vi "Handle Debug Data.vi"(8 "error in (no error)":errorcluster, 10 "Debug Data.lvclass":refnum<class "Debug Data.lvclass">, 11 "Debug Data Event In":refnum<class "Mock Data Listener.lvclass">) -> (0 "error out":errorcluster, 3 "Debug Data Event Out":refnum<class "Mock Data Listener.lvclass">)   [LabVIEW 2020, in "Mock Data Listener.lvclass"]
uses:
  Mock Data Listener.lvclass
  Debug Data/Debug Data.lvclass
  Mock Data Listener.lvclass/Mock Data Listener.ctl
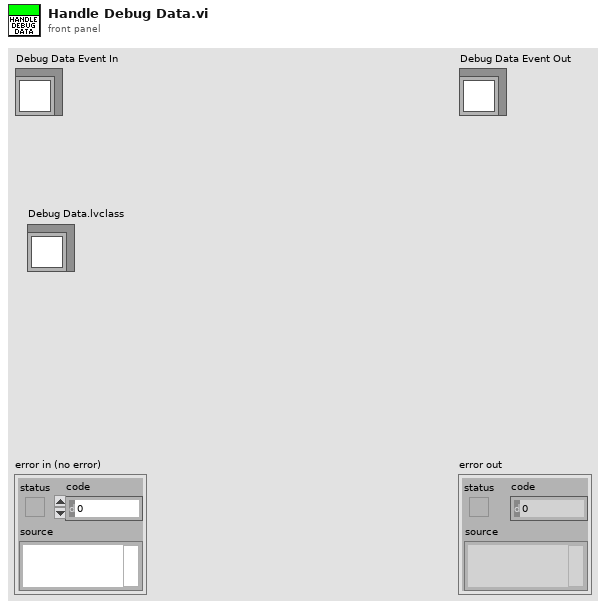
[diagram p1: front panel]
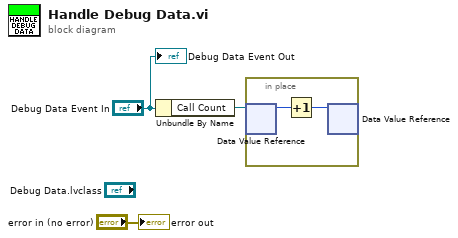
[diagram p0: block diagram]
diagram:
  n1 = Unbundle By Name("Debug Data Event In") -> ("Call Count"=w1:refnum<data-value>)
  n2 = in-place {
    n3 = in-place-dvr #1(w1) -> (w5:i32)  [unwired: 1 out]
    n4 = Increment(x=w5) -> (x+1=w4:i32)
    n5 = in-place-dvr #1(w4) -> ()  [unwired: 2 out]
  }
  "error out" <- "error in (no error)"
  "Debug Data Event Out" <- "Debug Data Event In"
